vi "Testwithoutvariants.vi"() -> ()   [LabVIEW 2024]
panel:
  out "Message Based Settings:Termination Character":u8
  out "OutPut":string
  out "error out":errorcluster
  in  "error in (no error)":errorcluster
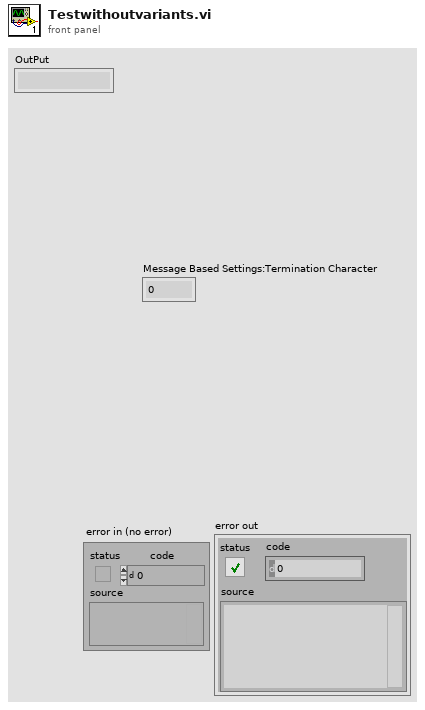
[diagram p1: front panel]
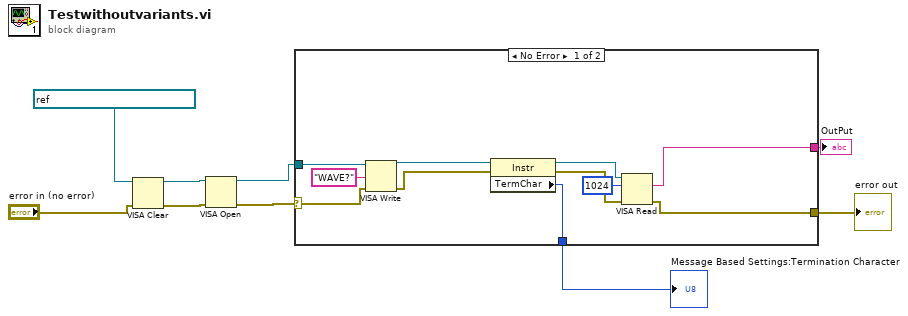
[diagram p0: block diagram]
diagram:
  n1 = VISA Clear(VISA resource name=refnum<visa-resource-name> "SaraMONOCHROMATOR", error in (no error)="error in (no error)") -> (VISA resource name out=w4:refnum<visa-resource-name>, error out=w3:errorcluster)
  n2 = VISA Open(error in (no error)=w3, VISA resource name=w4) -> (VISA resource name=w1:refnum<visa-resource-name>, error out=w2:errorcluster)  [unwired: 3 in]
  n3 = case shown="No Error" w2 {
    selector: w2 -> [w19 _]
    tunnel: [w20 _] -> w9
    tunnel: [w16 _] -> w8
    tunnel: [w14 _] -> w7
    tunnel: w1 -> [w10 _]
    frame No Error {
      n4 = VISA Write(VISA resource name=w10, write buffer="WAVE?", error in (no error)=w19) -> (VISA resource name out=w17:refnum<visa-resource-name>, error out=w13:errorcluster)  [unwired: 1 out]
      n5 = property class="Instr"(reference=w17, error in=w13) -> (reference out=w15:refnum<visa-resource-name>, error out=w12:errorcluster, "TermChar"=w14:u8)
      n6 = VISA Read(VISA resource name=w15, byte count=u32 1024, error in (no error)=w12) -> (read buffer=w20:string, error out=w16:errorcluster)  [unwired: 2 out]
    }
    frame Error {
    }
  }
  "OutPut" <- w9
  "error out" <- w8
  "Message Based Settings:Termination Character" <- w7
